vi "Read Dates.vi"(1 "File Path":path, 4 "Calibration Due":T1 {"Eq20" format="%<%x>T"; "Eq19" format="%<%x>T"; "Eq18" format="%<%x>T"; "Eq17" format="%<%x>T"; "Eq16" format="%<%x>T"; "Eq15" format="%<%x>T"; "Eq14" format="%<%x>T"; "Eq13" format="%<%x>T"; "Eq12" format="%<%x>T"; "Eq11" format="%<%x>T"; "Eq10" format="%<%x>T"; "Eq9" format="%<%x>T"; "Eq8" format="%<%x>T"; "Eq7" format="%<%x>T"; "Eq6" format="%<%x>T"; "Eq5" format="%<%x>T"; "Eq4" format="%<%x>T"; "Eq3" format="%<%x>T"; "Eq2" format="%<%x>T"; "Eq1" format="%<%x>T"}, 5 "Last Calibrated":T1 {"Eq20" format="%<%x>T"; "Eq19" format="%<%x>T"; "Eq18" format="%<%x>T"; "Eq17" format="%<%x>T"; "Eq16" format="%<%x>T"; "Eq15" format="%<%x>T"; "Eq14" format="%<%x>T"; "Eq13" format="%<%x>T"; "Eq12" format="%<%x>T"; "Eq11" format="%<%x>T"; "Eq10" format="%<%x>T"; "Eq9" format="%<%x>T"; "Eq8" format="%<%x>T"; "Eq7" format="%<%x>T"; "Eq6" format="%<%x>T"; "Eq5" format="%<%x>T"; "Eq4" format="%<%x>T"; "Eq3" format="%<%x>T"; "Eq2" format="%<%x>T"; "Eq1" format="%<%x>T"}, 6 "Serial Number":T2, 7 "Calibration ID":T3, 8 "error in (no error)":errorcluster, 9 "Model Number":T3, 10 "Manufacturer":T3, 11 "Equipment Description":T3) -> (0 "error out":errorcluster, 3 "output cluster":T4 {"Calibration Due"."Eq20" format="%<%x>T"; "Calibration Due"."Eq19" format="%<%x>T"; "Calibration Due"."Eq18" format="%<%x>T"; "Calibration Due"."Eq17" format="%<%x>T"; "Calibration Due"."Eq16" format="%<%x>T"; "Calibration Due"."Eq15" format="%<%x>T"; "Calibration Due"."Eq14" format="%<%x>T"; "Calibration Due"."Eq13" format="%<%x>T"; "Calibration Due"."Eq12" format="%<%x>T"; "Calibration Due"."Eq11" format="%<%x>T"; "Calibration Due"."Eq10" format="%<%x>T"; "Calibration Due"."Eq9" format="%<%x>T"; "Calibration Due"."Eq8" format="%<%x>T"; "Calibration Due"."Eq7" format="%<%x>T"; "Calibration Due"."Eq6" format="%<%x>T"; "Calibration Due"."Eq5" format="%<%x>T"; "Calibration Due"."Eq4" format="%<%x>T"; "Calibration Due"."Eq3" format="%<%x>T"; "Calibration Due"."Eq2" format="%<%x>T"; "Calibration Due"."Eq1" format="%<%x>T"; "Last Calibrated"."Eq20" format="%<%x>T"; "Last Calibrated"."Eq19" format="%<%x>T"; "Last Calibrated"."Eq18" format="%<%x>T"; "Last Calibrated"."Eq17" format="%<%x>T"; "Last Calibrated"."Eq16" format="%<%x>T"; "Last Calibrated"."Eq15" format="%<%x>T"; "Last Calibrated"."Eq14" format="%<%x>T"; "Last Calibrated"."Eq13" format="%<%x>T"; "Last Calibrated"."Eq12" format="%<%x>T"; "Last Calibrated"."Eq11" format="%<%x>T"; "Last Calibrated"."Eq10" format="%<%x>T"; "Last Calibrated"."Eq9" format="%<%x>T"; "Last Calibrated"."Eq8" format="%<%x>T"; "Last Calibrated"."Eq7" format="%<%x>T"; "Last Calibrated"."Eq6" format="%<%x>T"; "Last Calibrated"."Eq5" format="%<%x>T"; "Last Calibrated"."Eq4" format="%<%x>T"; "Last Calibrated"."Eq3" format="%<%x>T"; "Last Calibrated"."Eq2" format="%<%x>T"; "Last Calibrated"."Eq1" format="%<%x>T"})   [LabVIEW 2012]
uses:
  CalibrationTime.ctl
  Calibration.ctl
  Calibration_SN.ctl
  <vilib>/Utility/file.llb/Read From Spreadsheet File (string).vi
panel:
  in  "Tab Control":enum32{"Controls", "Read Data"}(tab)
  out "Equipment Description":T3
  out "Manufacturer":T3
  out "Model Number":T3
  out "Last Calibrated":T1 {"Eq20" format="%<%x>T"; "Eq19" format="%<%x>T"; "Eq18" format="%<%x>T"; "Eq17" format="%<%x>T"; "Eq16" format="%<%x>T"; "Eq15" format="%<%x>T"; "Eq14" format="%<%x>T"; "Eq13" format="%<%x>T"; "Eq12" format="%<%x>T"; "Eq11" format="%<%x>T"; "Eq10" format="%<%x>T"; "Eq9" format="%<%x>T"; "Eq8" format="%<%x>T"; "Eq7" format="%<%x>T"; "Eq6" format="%<%x>T"; "Eq5" format="%<%x>T"; "Eq4" format="%<%x>T"; "Eq3" format="%<%x>T"; "Eq2" format="%<%x>T"; "Eq1" format="%<%x>T"}
  out "Serial Number":T2
  out "Calibration ID.":T3
  out "Calibration Due":T1 {"Eq20" format="%<%x>T"; "Eq19" format="%<%x>T"; "Eq18" format="%<%x>T"; "Eq17" format="%<%x>T"; "Eq16" format="%<%x>T"; "Eq15" format="%<%x>T"; "Eq14" format="%<%x>T"; "Eq13" format="%<%x>T"; "Eq12" format="%<%x>T"; "Eq11" format="%<%x>T"; "Eq10" format="%<%x>T"; "Eq9" format="%<%x>T"; "Eq8" format="%<%x>T"; "Eq7" format="%<%x>T"; "Eq6" format="%<%x>T"; "Eq5" format="%<%x>T"; "Eq4" format="%<%x>T"; "Eq3" format="%<%x>T"; "Eq2" format="%<%x>T"; "Eq1" format="%<%x>T"}
  out "Size":i32
  out "all rows":string[][](array[string])
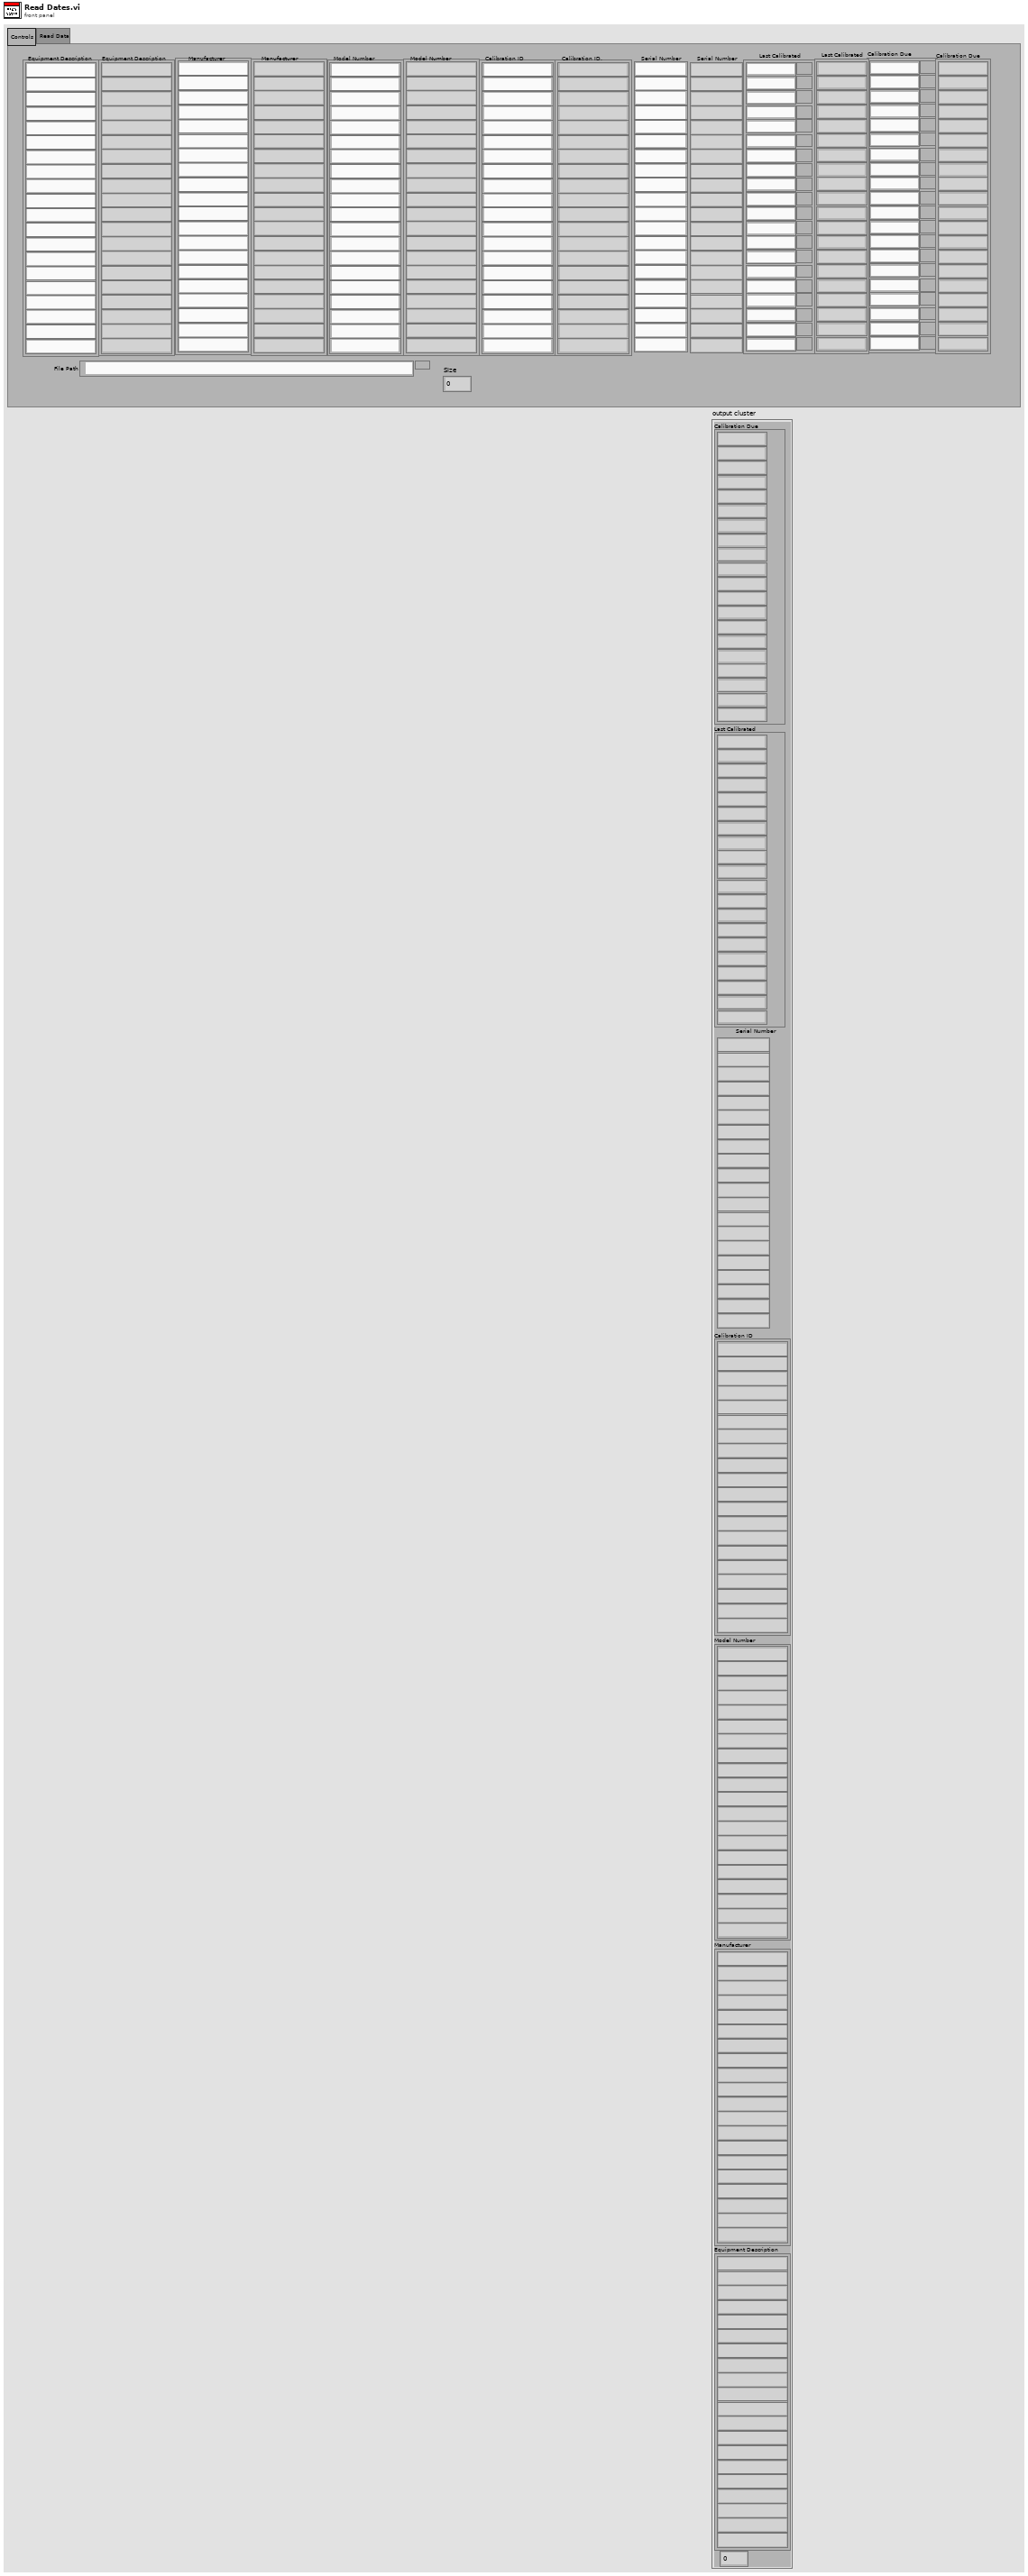
[diagram p1: front panel]
types:
  T1 = typedef "CalibrationTime.ctl" = cluster{"Eq1":timestamp, "Eq2":timestamp, "Eq3":timestamp, "Eq4":timestamp, "Eq5":timestamp, "Eq6":timestamp, "Eq7":timestamp, "Eq8":timestamp, "Eq9":timestamp, "Eq10":timestamp, "Eq11":timestamp, "Eq12":timestamp, "Eq13":timestamp, "Eq14":timestamp, "Eq15":timestamp, "Eq16":timestamp, "Eq17":timestamp, "Eq18":timestamp, "Eq19":timestamp, "Eq20":timestamp}
  T2 = typedef "Calibration_SN.ctl" = cluster{"Eq1":string, "Eq2":string, "Eq3":string, "Eq4":string, "Eq5":string, "Eq6":string, "Eq7":string, "Eq8":string, "Eq9":string, "Eq10":string, "Eq11":string, "Eq12":string, "Eq13":string, "Eq14":string, "Eq15":string, "Eq16":string, "Eq17":string, "Eq18":string, "Eq19":string, "Eq20":string}
  T3 = typedef "Calibration.ctl" = cluster{"Eq1":string, "Eq2":string, "Eq3":string, "Eq4":string, "Eq5":string, "Eq6":string, "Eq7":string, "Eq8":string, "Eq9":string, "Eq10":string, "Eq11":string, "Eq12":string, "Eq13":string, "Eq14":string, "Eq15":string, "Eq16":string, "Eq17":string, "Eq18":string, "Eq19":string, "Eq20":string}
  T4 = cluster{"Calibration Due":T1, "Last Calibrated":T1, "Serial Number":T2, "Calibration ID":T3, "Model Number":T3, "Manufacturer":T3, "Equipment Description":T3, i32}
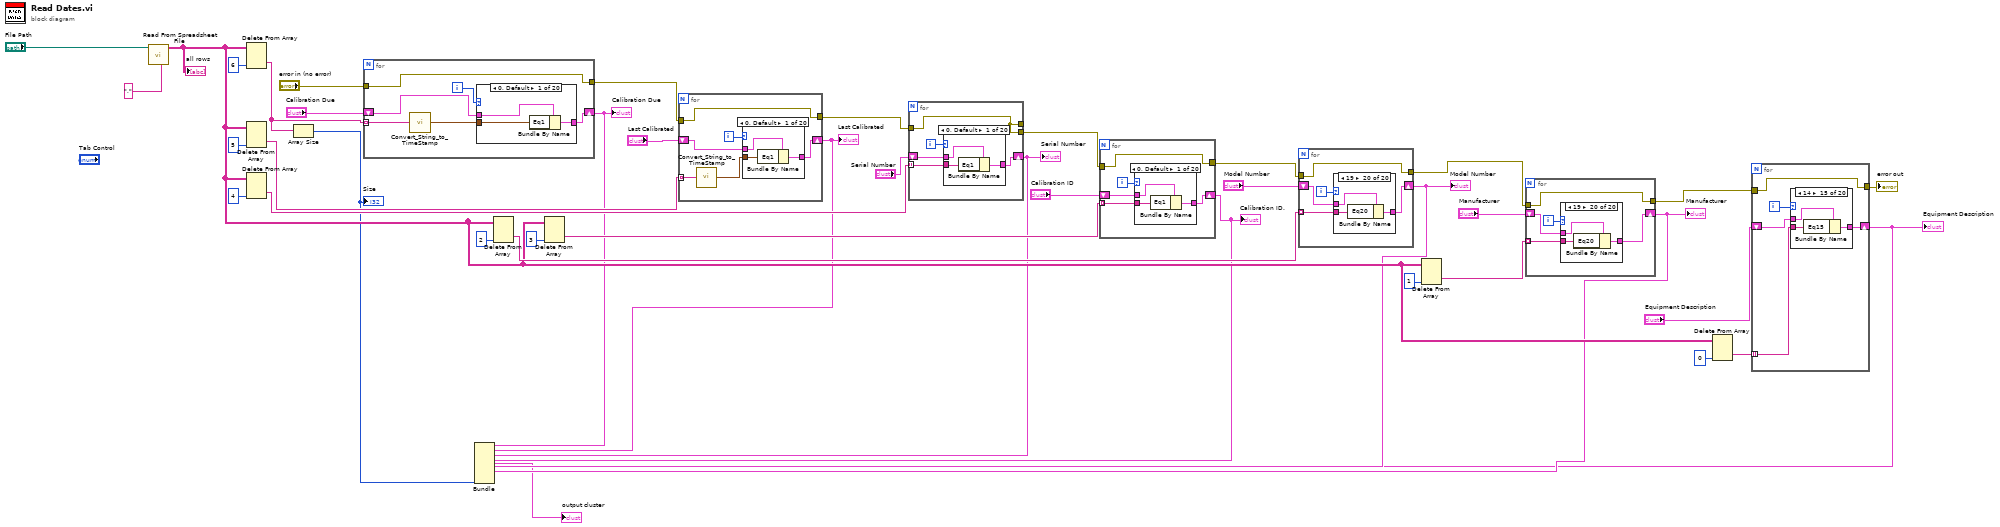
[diagram p0: block diagram]
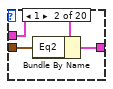
[diagram p2: hidden frame]
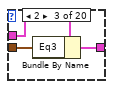
[diagram p3: hidden frame]
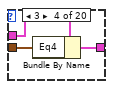
[diagram p4: hidden frame]
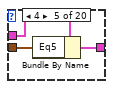
[diagram p5: hidden frame]
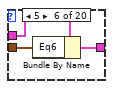
[diagram p6: hidden frame]
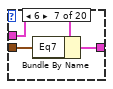
[diagram p7: hidden frame]
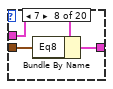
[diagram p8: hidden frame]
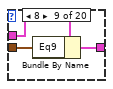
[diagram p9: hidden frame]
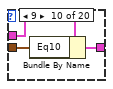
[diagram p10: hidden frame]
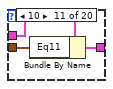
[diagram p11: hidden frame]
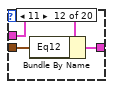
[diagram p12: hidden frame]
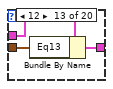
[diagram p13: hidden frame]
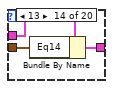
[diagram p14: hidden frame]
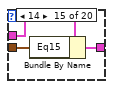
[diagram p15: hidden frame]
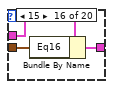
[diagram p16: hidden frame]
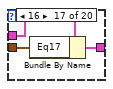
[diagram p17: hidden frame]
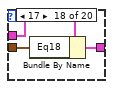
[diagram p18: hidden frame]
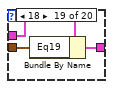
[diagram p19: hidden frame]
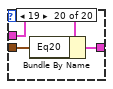
[diagram p20: hidden frame]
diagram:
  n1 = call-poly <vilib>:"Read From Spreadsheet File.vi"("delimiter (\\t)"="," ("delimiter (\\t)"), "file path (dialog if empty)"="File Path") -> ("all rows"=w13:string[][])  [unwired: 5 in, 4 out]
  "all rows" <- w13
  n2 = Delete From Array(array=w13, index (col)=6 ("disabled index (col)")) -> (deleted portion=w31:string[])  [unwired: 2 in, 1 out]
  n3 = Delete From Array(array=w13, index (col)=5 ("disabled index (col)")) -> (deleted portion=w11:string[])  [unwired: 2 in, 1 out]
  n4 = Delete From Array(array=w13, index (col)=4 ("disabled index (col)")) -> (deleted portion=w17:string[])  [unwired: 2 in, 1 out]
  n5 = Array Size(array=w31) -> (size(s)=w2:i32)
  "Size" <- w2
  n6 = for {
    tunnel: w31 -> [w47] mode=indexing
    shift-right: [w43] -> w9
    shift-left: "Calibration Due" -> [w45]
    tunnel: [w42] -> w15
    tunnel: "error in (no error)" -> [w42]
    i -> [w46]
    n7 = call "Convert_String_to_TimeStamp.vi"("date/time string"=w47) -> ("Resulting Time Stamp"=w44:timestamp)
    n8 = case shown="0, Default" w46 {
      tunnel: w45 -> [w49 w52 w55 w58 w61 w64 w67 w70 w73 w76 w79 w82 w85 w88 w92 w95 w98 w101 w103 w106]
      tunnel: w44 -> [w50 w53 w56 w59 w62 w65 w68 w71 w74 w77 w80 w83 w86 w89 w91 w94 w97 w99 w104 w107]
      tunnel: [w48 w51 w54 w57 w60 w63 w66 w69 w72 w75 w78 w81 w84 w87 w90 w93 w96 w100 w102 w105] -> w43
      frame 0, Default {
        n9 = Bundle By Name(cluster=w49, "Eq1"=w50) -> (w48:T1)
      }
      frame 1 {
        n10 = Bundle By Name(cluster=w52, "Eq2"=w53) -> (w51:T1)
      }
      frame 2 {
        n11 = Bundle By Name(cluster=w55, "Eq3"=w56) -> (w54:T1)
      }
      frame 3 {
        n12 = Bundle By Name(cluster=w58, "Eq4"=w59) -> (w57:T1)
      }
      frame 4 {
        n13 = Bundle By Name(cluster=w61, "Eq5"=w62) -> (w60:T1)
      }
      frame 5 {
        n14 = Bundle By Name(cluster=w64, "Eq6"=w65) -> (w63:T1)
      }
      frame 6 {
        n15 = Bundle By Name(cluster=w67, "Eq7"=w68) -> (w66:T1)
      }
      frame 7 {
        n16 = Bundle By Name(cluster=w70, "Eq8"=w71) -> (w69:T1)
      }
      frame 8 {
        n17 = Bundle By Name(cluster=w73, "Eq9"=w74) -> (w72:T1)
      }
      frame 9 {
        n18 = Bundle By Name(cluster=w76, "Eq10"=w77) -> (w75:T1)
      }
      frame 10 {
        n19 = Bundle By Name(cluster=w79, "Eq11"=w80) -> (w78:T1)
      }
      frame 11 {
        n20 = Bundle By Name(cluster=w82, "Eq12"=w83) -> (w81:T1)
      }
      frame 12 {
        n21 = Bundle By Name(cluster=w85, "Eq13"=w86) -> (w84:T1)
      }
      frame 13 {
        n22 = Bundle By Name(cluster=w88, "Eq14"=w89) -> (w87:T1)
      }
      frame 14 {
        n23 = Bundle By Name(cluster=w92, "Eq15"=w91) -> (w90:T1)
      }
      frame 15 {
        n24 = Bundle By Name(cluster=w95, "Eq16"=w94) -> (w93:T1)
      }
      frame 16 {
        n25 = Bundle By Name(cluster=w98, "Eq17"=w97) -> (w96:T1)
      }
      frame 17 {
        n26 = Bundle By Name(cluster=w101, "Eq18"=w99) -> (w100:T1)
      }
      frame 18 {
        n27 = Bundle By Name(cluster=w103, "Eq19"=w104) -> (w102:T1)
      }
      frame 19 {
        n28 = Bundle By Name(cluster=w106, "Eq20"=w107) -> (w105:T1)
      }
    }
  }
  "Calibration Due" <- w9
  n29 = Delete From Array(array=w13, index (col)=2 ("disabled index (col)")) -> (deleted portion=w33:string[])  [unwired: 2 in, 1 out]
  n30 = Delete From Array(array=w13, index (col)=3 ("disabled index (col)")) -> (deleted portion=w21:string[])  [unwired: 2 in, 1 out]
  n31 = for {
    tunnel: w11 -> [w113] mode=indexing
    shift-right: [w109] -> w8
    shift-left: "Last Calibrated" -> [w111]
    tunnel: [w108] -> w14
    tunnel: w15 -> [w108]
    i -> [w112]
    n32 = call "Convert_String_to_TimeStamp.vi"("date/time string"=w113) -> ("Resulting Time Stamp"=w110:timestamp)
    n33 = case shown="0, Default" w112 {
      tunnel: w111 -> [w115 w118 w121 w124 w127 w130 w133 w136 w139 w142 w145 w148 w151 w154 w158 w161 w164 w167 w169 w172]
      tunnel: w110 -> [w116 w119 w122 w125 w128 w131 w134 w137 w140 w143 w146 w149 w152 w155 w157 w160 w163 w165 w170 w173]
      tunnel: [w114 w117 w120 w123 w126 w129 w132 w135 w138 w141 w144 w147 w150 w153 w156 w159 w162 w166 w168 w171] -> w109
      frame 0, Default {
        n34 = Bundle By Name(cluster=w115, "Eq1"=w116) -> (w114:T1)
      }
      frame 1 {
        n35 = Bundle By Name(cluster=w118, "Eq2"=w119) -> (w117:T1)
      }
      frame 2 {
        n36 = Bundle By Name(cluster=w121, "Eq3"=w122) -> (w120:T1)
      }
      frame 3 {
        n37 = Bundle By Name(cluster=w124, "Eq4"=w125) -> (w123:T1)
      }
      frame 4 {
        n38 = Bundle By Name(cluster=w127, "Eq5"=w128) -> (w126:T1)
      }
      frame 5 {
        n39 = Bundle By Name(cluster=w130, "Eq6"=w131) -> (w129:T1)
      }
      frame 6 {
        n40 = Bundle By Name(cluster=w133, "Eq7"=w134) -> (w132:T1)
      }
      frame 7 {
        n41 = Bundle By Name(cluster=w136, "Eq8"=w137) -> (w135:T1)
      }
      frame 8 {
        n42 = Bundle By Name(cluster=w139, "Eq9"=w140) -> (w138:T1)
      }
      frame 9 {
        n43 = Bundle By Name(cluster=w142, "Eq10"=w143) -> (w141:T1)
      }
      frame 10 {
        n44 = Bundle By Name(cluster=w145, "Eq11"=w146) -> (w144:T1)
      }
      frame 11 {
        n45 = Bundle By Name(cluster=w148, "Eq12"=w149) -> (w147:T1)
      }
      frame 12 {
        n46 = Bundle By Name(cluster=w151, "Eq13"=w152) -> (w150:T1)
      }
      frame 13 {
        n47 = Bundle By Name(cluster=w154, "Eq14"=w155) -> (w153:T1)
      }
      frame 14 {
        n48 = Bundle By Name(cluster=w158, "Eq15"=w157) -> (w156:T1)
      }
      frame 15 {
        n49 = Bundle By Name(cluster=w161, "Eq16"=w160) -> (w159:T1)
      }
      frame 16 {
        n50 = Bundle By Name(cluster=w164, "Eq17"=w163) -> (w162:T1)
      }
      frame 17 {
        n51 = Bundle By Name(cluster=w167, "Eq18"=w165) -> (w166:T1)
      }
      frame 18 {
        n52 = Bundle By Name(cluster=w169, "Eq19"=w170) -> (w168:T1)
      }
      frame 19 {
        n53 = Bundle By Name(cluster=w172, "Eq20"=w173) -> (w171:T1)
      }
    }
  }
  "Last Calibrated" <- w8
  n54 = for {
    tunnel: w17 -> [w175] mode=indexing
    shift-right: [w176] -> w7
    shift-left: "Serial Number" -> [w177]
    tunnel: [w174] -> _
    tunnel: w14 -> [w174]
    tunnel: [w174] -> w19
    i -> [w178]
    n55 = case shown="0, Default" w178 {
      tunnel: w177 -> [w181 w184 w187 w190 w193 w196 w199 w202 w205 w208 w211 w214 w217 w220 w223 w226 w228 w231 w234 w237]
      tunnel: [w180 w183 w186 w189 w192 w195 w198 w201 w204 w207 w210 w213 w216 w219 w222 w224 w227 w230 w233 w236] -> w176
      tunnel: w175 -> [w179 w182 w185 w188 w191 w194 w197 w200 w203 w206 w209 w212 w215 w218 w221 w225 w229 w232 w235 w238]
      frame 0, Default {
        n56 = Bundle By Name(cluster=w181, "Eq1"=w179) -> (w180:T2)
      }
      frame 1 {
        n57 = Bundle By Name(cluster=w184, "Eq2"=w182) -> (w183:T2)
      }
      frame 2 {
        n58 = Bundle By Name(cluster=w187, "Eq3"=w185) -> (w186:T2)
      }
      frame 3 {
        n59 = Bundle By Name(cluster=w190, "Eq4"=w188) -> (w189:T2)
      }
      frame 4 {
        n60 = Bundle By Name(cluster=w193, "Eq5"=w191) -> (w192:T2)
      }
      frame 5 {
        n61 = Bundle By Name(cluster=w196, "Eq6"=w194) -> (w195:T2)
      }
      frame 6 {
        n62 = Bundle By Name(cluster=w199, "Eq7"=w197) -> (w198:T2)
      }
      frame 7 {
        n63 = Bundle By Name(cluster=w202, "Eq8"=w200) -> (w201:T2)
      }
      frame 8 {
        n64 = Bundle By Name(cluster=w205, "Eq9"=w203) -> (w204:T2)
      }
      frame 9 {
        n65 = Bundle By Name(cluster=w208, "Eq10"=w206) -> (w207:T2)
      }
      frame 10 {
        n66 = Bundle By Name(cluster=w211, "Eq11"=w209) -> (w210:T2)
      }
      frame 11 {
        n67 = Bundle By Name(cluster=w214, "Eq12"=w212) -> (w213:T2)
      }
      frame 12 {
        n68 = Bundle By Name(cluster=w217, "Eq13"=w215) -> (w216:T2)
      }
      frame 13 {
        n69 = Bundle By Name(cluster=w220, "Eq14"=w218) -> (w219:T2)
      }
      frame 14 {
        n70 = Bundle By Name(cluster=w223, "Eq15"=w221) -> (w222:T2)
      }
      frame 15 {
        n71 = Bundle By Name(cluster=w226, "Eq16"=w225) -> (w224:T2)
      }
      frame 16 {
        n72 = Bundle By Name(cluster=w228, "Eq17"=w229) -> (w227:T2)
      }
      frame 17 {
        n73 = Bundle By Name(cluster=w231, "Eq18"=w232) -> (w230:T2)
      }
      frame 18 {
        n74 = Bundle By Name(cluster=w234, "Eq19"=w235) -> (w233:T2)
      }
      frame 19 {
        n75 = Bundle By Name(cluster=w237, "Eq20"=w238) -> (w236:T2)
      }
    }
  }
  "Serial Number" <- w7
  n76 = for {
    tunnel: w21 -> [w239] mode=indexing
    shift-right: [w241] -> w6
    shift-left: "Calibration ID" -> [w242]
    tunnel: [w240] -> w22
    tunnel: w19 -> [w240]
    i -> [w243]
    n77 = case shown="0, Default" w243 {
      tunnel: w242 -> [w246 w249 w252 w255 w258 w261 w264 w267 w270 w273 w276 w279 w282 w285 w288 w291 w293 w296 w299 w302]
      tunnel: [w245 w248 w251 w254 w257 w260 w263 w266 w269 w272 w275 w278 w281 w284 w287 w289 w292 w295 w298 w301] -> w241
      tunnel: w239 -> [w244 w247 w250 w253 w256 w259 w262 w265 w268 w271 w274 w277 w280 w283 w286 w290 w294 w297 w300 w303]
      frame 0, Default {
        n78 = Bundle By Name(cluster=w246, "Eq1"=w244) -> (w245:T3)
      }
      frame 1 {
        n79 = Bundle By Name(cluster=w249, "Eq2"=w247) -> (w248:T3)
      }
      frame 2 {
        n80 = Bundle By Name(cluster=w252, "Eq3"=w250) -> (w251:T3)
      }
      frame 3 {
        n81 = Bundle By Name(cluster=w255, "Eq4"=w253) -> (w254:T3)
      }
      frame 4 {
        n82 = Bundle By Name(cluster=w258, "Eq5"=w256) -> (w257:T3)
      }
      frame 5 {
        n83 = Bundle By Name(cluster=w261, "Eq6"=w259) -> (w260:T3)
      }
      frame 6 {
        n84 = Bundle By Name(cluster=w264, "Eq7"=w262) -> (w263:T3)
      }
      frame 7 {
        n85 = Bundle By Name(cluster=w267, "Eq8"=w265) -> (w266:T3)
      }
      frame 8 {
        n86 = Bundle By Name(cluster=w270, "Eq9"=w268) -> (w269:T3)
      }
      frame 9 {
        n87 = Bundle By Name(cluster=w273, "Eq10"=w271) -> (w272:T3)
      }
      frame 10 {
        n88 = Bundle By Name(cluster=w276, "Eq11"=w274) -> (w275:T3)
      }
      frame 11 {
        n89 = Bundle By Name(cluster=w279, "Eq12"=w277) -> (w278:T3)
      }
      frame 12 {
        n90 = Bundle By Name(cluster=w282, "Eq13"=w280) -> (w281:T3)
      }
      frame 13 {
        n91 = Bundle By Name(cluster=w285, "Eq14"=w283) -> (w284:T3)
      }
      frame 14 {
        n92 = Bundle By Name(cluster=w288, "Eq15"=w286) -> (w287:T3)
      }
      frame 15 {
        n93 = Bundle By Name(cluster=w291, "Eq16"=w290) -> (w289:T3)
      }
      frame 16 {
        n94 = Bundle By Name(cluster=w293, "Eq17"=w294) -> (w292:T3)
      }
      frame 17 {
        n95 = Bundle By Name(cluster=w296, "Eq18"=w297) -> (w295:T3)
      }
      frame 18 {
        n96 = Bundle By Name(cluster=w299, "Eq19"=w300) -> (w298:T3)
      }
      frame 19 {
        n97 = Bundle By Name(cluster=w302, "Eq20"=w303) -> (w301:T3)
      }
    }
  }
  "Calibration ID." <- w6
  n98 = for {
    tunnel: w33 -> [w304] mode=indexing
    shift-right: [w306] -> w5
    shift-left: "Model Number" -> [w307]
    tunnel: [w305] -> w37
    tunnel: w22 -> [w305]
    i -> [w308]
    n99 = case shown="19" w308 {
      tunnel: w307 -> [w311 w314 w317 w320 w323 w326 w329 w332 w335 w338 w341 w344 w347 w350 w353 w356 w358 w361 w364 w367]
      tunnel: [w310 w313 w316 w319 w322 w325 w328 w331 w334 w337 w340 w343 w346 w349 w352 w354 w357 w360 w363 w366] -> w306
      tunnel: w304 -> [w309 w312 w315 w318 w321 w324 w327 w330 w333 w336 w339 w342 w345 w348 w351 w355 w359 w362 w365 w368]
      frame 0, Default {
        n100 = Bundle By Name(cluster=w311, "Eq1"=w309) -> (w310:T3)
      }
      frame 1 {
        n101 = Bundle By Name(cluster=w314, "Eq2"=w312) -> (w313:T3)
      }
      frame 2 {
        n102 = Bundle By Name(cluster=w317, "Eq3"=w315) -> (w316:T3)
      }
      frame 3 {
        n103 = Bundle By Name(cluster=w320, "Eq4"=w318) -> (w319:T3)
      }
      frame 4 {
        n104 = Bundle By Name(cluster=w323, "Eq5"=w321) -> (w322:T3)
      }
      frame 5 {
        n105 = Bundle By Name(cluster=w326, "Eq6"=w324) -> (w325:T3)
      }
      frame 6 {
        n106 = Bundle By Name(cluster=w329, "Eq7"=w327) -> (w328:T3)
      }
      frame 7 {
        n107 = Bundle By Name(cluster=w332, "Eq8"=w330) -> (w331:T3)
      }
      frame 8 {
        n108 = Bundle By Name(cluster=w335, "Eq9"=w333) -> (w334:T3)
      }
      frame 9 {
        n109 = Bundle By Name(cluster=w338, "Eq10"=w336) -> (w337:T3)
      }
      frame 10 {
        n110 = Bundle By Name(cluster=w341, "Eq11"=w339) -> (w340:T3)
      }
      frame 11 {
        n111 = Bundle By Name(cluster=w344, "Eq12"=w342) -> (w343:T3)
      }
      frame 12 {
        n112 = Bundle By Name(cluster=w347, "Eq13"=w345) -> (w346:T3)
      }
      frame 13 {
        n113 = Bundle By Name(cluster=w350, "Eq14"=w348) -> (w349:T3)
      }
      frame 14 {
        n114 = Bundle By Name(cluster=w353, "Eq15"=w351) -> (w352:T3)
      }
      frame 15 {
        n115 = Bundle By Name(cluster=w356, "Eq16"=w355) -> (w354:T3)
      }
      frame 16 {
        n116 = Bundle By Name(cluster=w358, "Eq17"=w359) -> (w357:T3)
      }
      frame 17 {
        n117 = Bundle By Name(cluster=w361, "Eq18"=w362) -> (w360:T3)
      }
      frame 18 {
        n118 = Bundle By Name(cluster=w364, "Eq19"=w365) -> (w363:T3)
      }
      frame 19 {
        n119 = Bundle By Name(cluster=w367, "Eq20"=w368) -> (w366:T3)
      }
    }
  }
  "Model Number" <- w5
  n120 = Delete From Array(array=w13, index (col)=1 ("disabled index (col)")) -> (deleted portion=w32:string[])  [unwired: 2 in, 1 out]
  n121 = for {
    tunnel: w32 -> [w369] mode=indexing
    shift-right: [w371] -> w4
    shift-left: "Manufacturer" -> [w372]
    tunnel: [w370] -> w27
    tunnel: w37 -> [w370]
    i -> [w373]
    n122 = case shown="19" w373 {
      tunnel: w372 -> [w375 w378 w381 w384 w387 w390 w393 w396 w399 w402 w405 w408 w411 w414 w418 w420 w423 w426 w429 w432]
      tunnel: w369 -> [w376 w379 w382 w385 w388 w391 w394 w397 w400 w403 w406 w409 w412 w415 w417 w421 w424 w427 w430 w433]
      tunnel: [w374 w377 w380 w383 w386 w389 w392 w395 w398 w401 w404 w407 w410 w413 w416 w419 w422 w425 w428 w431] -> w371
      frame 0, Default {
        n123 = Bundle By Name(cluster=w375, "Eq1"=w376) -> (w374:T3)
      }
      frame 1 {
        n124 = Bundle By Name(cluster=w378, "Eq2"=w379) -> (w377:T3)
      }
      frame 2 {
        n125 = Bundle By Name(cluster=w381, "Eq3"=w382) -> (w380:T3)
      }
      frame 3 {
        n126 = Bundle By Name(cluster=w384, "Eq4"=w385) -> (w383:T3)
      }
      frame 4 {
        n127 = Bundle By Name(cluster=w387, "Eq5"=w388) -> (w386:T3)
      }
      frame 5 {
        n128 = Bundle By Name(cluster=w390, "Eq6"=w391) -> (w389:T3)
      }
      frame 6 {
        n129 = Bundle By Name(cluster=w393, "Eq7"=w394) -> (w392:T3)
      }
      frame 7 {
        n130 = Bundle By Name(cluster=w396, "Eq8"=w397) -> (w395:T3)
      }
      frame 8 {
        n131 = Bundle By Name(cluster=w399, "Eq9"=w400) -> (w398:T3)
      }
      frame 9 {
        n132 = Bundle By Name(cluster=w402, "Eq10"=w403) -> (w401:T3)
      }
      frame 10 {
        n133 = Bundle By Name(cluster=w405, "Eq11"=w406) -> (w404:T3)
      }
      frame 11 {
        n134 = Bundle By Name(cluster=w408, "Eq12"=w409) -> (w407:T3)
      }
      frame 12 {
        n135 = Bundle By Name(cluster=w411, "Eq13"=w412) -> (w410:T3)
      }
      frame 13 {
        n136 = Bundle By Name(cluster=w414, "Eq14"=w415) -> (w413:T3)
      }
      frame 14 {
        n137 = Bundle By Name(cluster=w418, "Eq15"=w417) -> (w416:T3)
      }
      frame 15 {
        n138 = Bundle By Name(cluster=w420, "Eq16"=w421) -> (w419:T3)
      }
      frame 16 {
        n139 = Bundle By Name(cluster=w423, "Eq17"=w424) -> (w422:T3)
      }
      frame 17 {
        n140 = Bundle By Name(cluster=w426, "Eq18"=w427) -> (w425:T3)
      }
      frame 18 {
        n141 = Bundle By Name(cluster=w429, "Eq19"=w430) -> (w428:T3)
      }
      frame 19 {
        n142 = Bundle By Name(cluster=w432, "Eq20"=w433) -> (w431:T3)
      }
    }
  }
  "Manufacturer" <- w4
  n143 = Delete From Array(array=w13, index (col)=0 ("disabled index (col)")) -> (deleted portion=w29:string[])  [unwired: 2 in, 1 out]
  n144 = for {
    tunnel: w29 -> [w434] mode=indexing
    shift-right: [w436] -> w3
    shift-left: "Equipment Description" -> [w437]
    tunnel: [w435] -> w26
    tunnel: w27 -> [w435]
    i -> [w438]
    n145 = case shown="14" w438 {
      tunnel: w437 -> [w440 w443 w446 w449 w452 w455 w458 w461 w464 w467 w470 w473 w476 w479 w483 w485 w488 w491 w494 w497]
      tunnel: w434 -> [w441 w444 w447 w450 w453 w456 w459 w462 w465 w468 w471 w474 w477 w480 w482 w486 w489 w492 w495 w498]
      tunnel: [w439 w442 w445 w448 w451 w454 w457 w460 w463 w466 w469 w472 w475 w478 w481 w484 w487 w490 w493 w496] -> w436
      frame 0, Default {
        n146 = Bundle By Name(cluster=w440, "Eq1"=w441) -> (w439:T3)
      }
      frame 1 {
        n147 = Bundle By Name(cluster=w443, "Eq2"=w444) -> (w442:T3)
      }
      frame 2 {
        n148 = Bundle By Name(cluster=w446, "Eq3"=w447) -> (w445:T3)
      }
      frame 3 {
        n149 = Bundle By Name(cluster=w449, "Eq4"=w450) -> (w448:T3)
      }
      frame 4 {
        n150 = Bundle By Name(cluster=w452, "Eq5"=w453) -> (w451:T3)
      }
      frame 5 {
        n151 = Bundle By Name(cluster=w455, "Eq6"=w456) -> (w454:T3)
      }
      frame 6 {
        n152 = Bundle By Name(cluster=w458, "Eq7"=w459) -> (w457:T3)
      }
      frame 7 {
        n153 = Bundle By Name(cluster=w461, "Eq8"=w462) -> (w460:T3)
      }
      frame 8 {
        n154 = Bundle By Name(cluster=w464, "Eq9"=w465) -> (w463:T3)
      }
      frame 9 {
        n155 = Bundle By Name(cluster=w467, "Eq10"=w468) -> (w466:T3)
      }
      frame 10 {
        n156 = Bundle By Name(cluster=w470, "Eq11"=w471) -> (w469:T3)
      }
      frame 11 {
        n157 = Bundle By Name(cluster=w473, "Eq12"=w474) -> (w472:T3)
      }
      frame 12 {
        n158 = Bundle By Name(cluster=w476, "Eq13"=w477) -> (w475:T3)
      }
      frame 13 {
        n159 = Bundle By Name(cluster=w479, "Eq14"=w480) -> (w478:T3)
      }
      frame 14 {
        n160 = Bundle By Name(cluster=w483, "Eq15"=w482) -> (w481:T3)
      }
      frame 15 {
        n161 = Bundle By Name(cluster=w485, "Eq16"=w486) -> (w484:T3)
      }
      frame 16 {
        n162 = Bundle By Name(cluster=w488, "Eq17"=w489) -> (w487:T3)
      }
      frame 17 {
        n163 = Bundle By Name(cluster=w491, "Eq18"=w492) -> (w490:T3)
      }
      frame 18 {
        n164 = Bundle By Name(cluster=w494, "Eq19"=w495) -> (w493:T3)
      }
      frame 19 {
        n165 = Bundle By Name(cluster=w497, "Eq20"=w498) -> (w496:T3)
      }
    }
  }
  "error out" <- w26
  "Equipment Description" <- w3
  n166 = Bundle("Calibration Due"=w9, "Last Calibrated"=w8, "Serial Number"=w7, "Calibration ID"=w6, "Model Number"=w5, "Manufacturer"=w4, "Equipment Description"=w3, w2) -> (→"output cluster":T4)  [unwired: 1 in]
